vi "I-V to Waveform parameters.vi"(4 "CIC filter factor":dbl=4.0 format="%#_13g", 6 "Input scale":dbl=3.0517577442878974e-05, 9 "Input range":dbl=1.0 format="%#_6p", 10 "Full output  bit range":i32=8192 format="0x%x (%d)", 11 "I-V parameters":T1={"Start magnitude"=0.001, "Magnitude increment"=0.001, "End magnitude"=7.0, "Ramp length"=32, "Top  length"=480, "Threshold "=0.0001, "Processing delay"=255, "Output gain "=0.01, "Interpolation"=64, "Stop after"=1, "Detector window"=480} {"Detector window" format="%dpts"; "Stop after" format="%d sweep(s)"; "Output gain" format="%#_6pA/V"; "Processing delay" format="%dpts"; "Threshold" format="%#_6pV"; "Top  length" format="%dpts"; "Ramp length" format="%dpts"; "End magnitude" format="%#_6pA"; "Magnitude increment" format="%#_6pA"; "Start magnitude" format="%#_6pA"}) -> (3 "Waveform parameters out":T2={"Start magnitude"=1000.0, "Magnitude increment"=500.0, "Number of pulses"=8, "Ramp length"=32, "Top  length"=480, "Threshold "=15729, "Processing delay"=240, "Stop after"=1, "Detector window"=480, "Upper limit"=8191, "Lower limit"=-8192} {"Lower limit" format="%d (0x%x)"; "Upper limit" format="%d (0x%x)"; "Detector window" format="%dpts"; "Stop after" format="%d sweep(s)"})   [LabVIEW 2021]
uses:
  Waveform parameters.ctl
  I-V parameters.ctl
panel:
  out "x/y":dbl
  out "End In Range?":bool
  out "Start In Range?":bool
  # "Waveform parameters"
  # "Detector parameters"
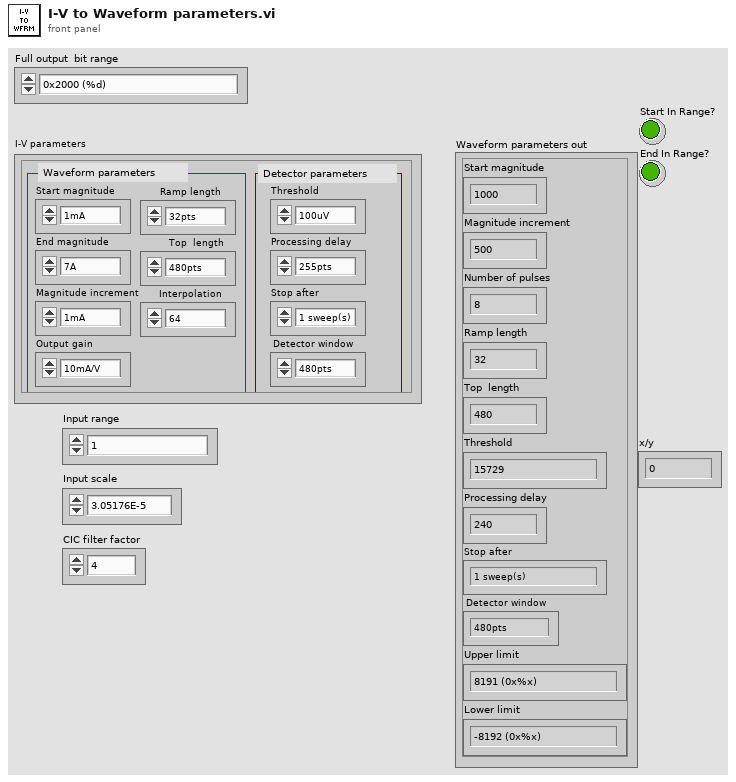
[diagram p1: front panel]
types:
  T1 = typedef "I-V parameters.ctl" = cluster{"Start magnitude":dbl, "Magnitude increment":dbl, "End magnitude":dbl, "Ramp length":i32, "Top  length":i32, "Threshold ":dbl, "Processing delay":u16, "Output gain ":dbl, "Interpolation":i32, "Stop after":u16, "Detector window":i32}
  T2 = typedef "Waveform parameters.ctl" = cluster{"Start magnitude":dbl, "Magnitude increment":dbl, "Number of pulses":i32, "Ramp length":i32, "Top  length":i32, "Threshold ":i32, "Processing delay":u16, "Stop after":u16, "Detector window":i32, "Upper limit":i16, "Lower limit":i16}
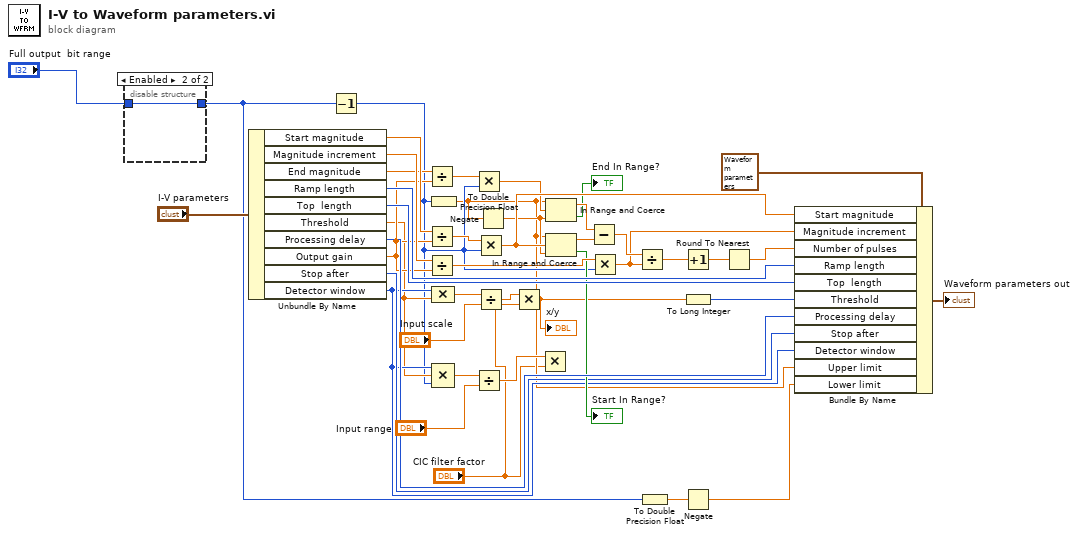
[diagram p0: block diagram]
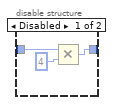
[diagram p2: hidden frame]
diagram:
  n1 = disable-structure shown="Enabled" {
    disable-tunnel: "Full output  bit range" -> [w46 w47]
    disable-tunnel: [w45 w47] -> w6
    frame Disabled {
      n2 = Multiply(x=w46, y=4) -> (x*y=w45:i32)
    }
    frame Enabled {
    }
  }
  n3 = Unbundle By Name("I-V parameters") -> ("Start magnitude"=w30:dbl, "Magnitude increment"=w33:dbl, "End magnitude"=w27:dbl, "Ramp length"=w40:i32, "Top  length"=w39:i32, "Threshold"=w12:dbl, "Processing delay"=w35:u16, "Output gain"=w20:dbl, "Stop after"=w14:u16, "Detector window"=w13:i32)
  n4 = Decrement(x=w6) -> (x-1=w9:i32)
  n5 = Divide(x=w27, y=w20) -> (x/y=w21:dbl)
  n6 = Divide(x=w30, y=w20) -> (x/y=w32:dbl)
  n7 = Divide(x=w33, y=w20) -> (x/y=w34:dbl)
  n8 = To Double Precision Float(number=w9) -> (double precision float=w8:dbl)
  n9 = Compound Arithmetic op=MULTIPLY(w13, w12) -> (w11:dbl)
  n10 = Compound Arithmetic op=MULTIPLY(w13, w12, w9) -> (w38:dbl)
  n11 = Multiply(x=w21, y=w9) -> (x*y=w19:dbl)
  n12 = Divide(x=w38, y="Input range") -> (x/y=w31:dbl)
  n13 = Multiply(x=w32, y=w9) -> (x*y=w28:dbl)
  n14 = Divide(x=w11, y="Input scale") -> (x/y=w2:dbl)
  n15 = Negate(x=w8) -> (-x=w26:dbl)
  n16 = Multiply(x=w2, y="CIC filter factor") -> (x*y=w1:dbl)
  "x/y" <- w1
  n17 = Multiply(x=w31, y="CIC filter factor") -> ()  [unwired: 1 out]
  n18 = In Range and Coerce(upper limit=w8, x=w19, lower limit=w26) -> (coerced(x)=w25:dbl, In Range?=→"End In Range?":bool)
  n19 = In Range and Coerce(upper limit=w8, x=w28, lower limit=w26) -> (coerced(x)=w24:dbl, In Range?=→"Start In Range?":bool)
  n20 = Subtract(x=w25, y=w24) -> (x-y=w16:dbl)
  n21 = Multiply(x=w34, y=w9) -> (x*y=w15:dbl)
  n22 = Divide(x=w16, y=w15) -> (x/y=w17:dbl)
  n23 = To Double Precision Float(number=w6) -> (double precision float=w5:dbl)
  n24 = Increment(x=w17) -> (x+1=w4:dbl)
  n25 = To Long Integer(number=w1) -> (32bit integer=w36:i32)
  n26 = Negate(x=w5) -> (-x=w7:dbl)
  n27 = Round To Nearest(number=w4) -> (nearest integer value=w29:dbl)
  n28 = Bundle By Name(cluster=T2 {"Start magnitude"=1000.0, "Magnitude increment"=500.0, "Number of pulses"=8, "Ramp length"=32, "Top  length"=480, "Threshold "=3000, "Processing delay"=240, "Stop after"=1, "Detector window"=480, "Upper limit"=32767, "Lower limit"=32767} ("Waveform parameters out"), "Start magnitude"=w28, "Magnitude increment"=w15, "Number of pulses"=w29, "Ramp length"=w40, "Top  length"=w39, "Threshold"=w36, "Processing delay"=w35, "Stop after"=w14, "Detector window"=w13, "Upper limit"=w8, "Lower limit"=w7) -> (→"Waveform parameters out":T2)
